vi "Connect PV.vi"(8 "error in (no error)":errorcluster, 10 "PV URL":string, 11 "CS++SVMonitor in":refnum<class "CS++SVMonitor.lvclass">) -> (0 "error out":errorcluster, 3 "CS++SVMonitor out":refnum<class "CS++SVMonitor.lvclass">)   [LabVIEW 2015, in "CS++SVMonitor.lvlib" / "CS++SVMonitor.lvclass"]
doc: "Open connection to process variable."
uses:
  CS++SVMonitor.lvclass
  CS++SVMonitor.lvclass/CS++SVMonitor.ctl
  Libraries/Utilities/CS++Utilities.lvlib
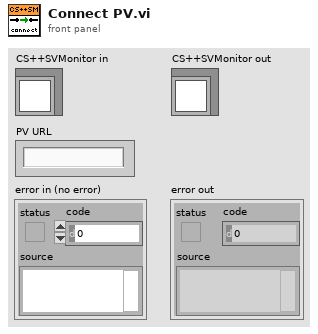
[diagram p1: front panel]
types:
  T1 = cluster{"Read Access":enum8{"Allowed", "Required", "None"}, "Write Access":enum8{"Allowed", "Required", "None"}}
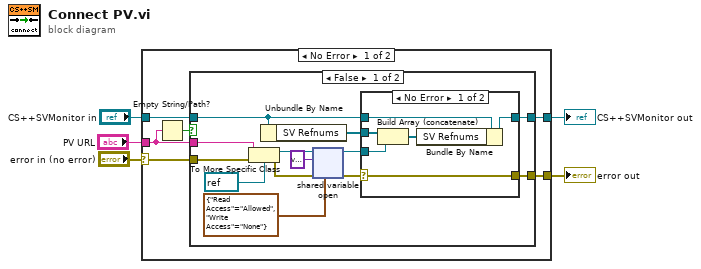
[diagram p0: block diagram]
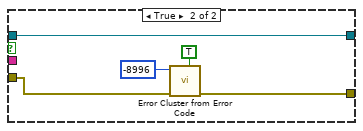
[diagram p3: hidden frame]
diagram:
  n1 = case shown="No Error" "error in (no error)" {
    selector: "error in (no error)" -> [w11 w39]
    tunnel: [w8 w39] -> w2
    tunnel: [w9 w38] -> w3
    tunnel: "CS++SVMonitor in" -> [w10 w38]
    tunnel: "PV URL" -> [w7 _]
    frame No Error {
      n2 = Empty String/Path?(string/path=w7) -> (empty?=w6:bool)
      n3 = case shown="False" w6 {
        tunnel: w11 -> [w19 w35]
        tunnel: w7 -> [w18 _]
        tunnel: w10 -> [w17 w37]
        tunnel: [w16 w37] -> w9
        tunnel: [w13 w34] -> w8
        frame False {
          n4 = To More Specific Class(target class=refnum<k21> refnum ("shared variable refnum in"), reference=w18, error in=w19) -> (specific class reference=w23:refnum<k21>, error out=w22:errorcluster)
          n5 = Unbundle By Name(w17) -> ("SV Refnums"=w15:refnum<k21>[])
          n6 = shared-variable-open(w23, w22, variant ("variant"), T1 {"Read Access"=enum."Allowed", "Write Access"=enum."None"} ("Access (R/W allowed)")) -> (w20:refnum<k21>, w14:errorcluster)
          n7 = case shown="No Error" w14 {
            selector: w14 -> [w25 w31]
            tunnel: w20 -> [w30 _]
            tunnel: w17 -> [w29 w32]
            tunnel: [w28 w32] -> w16
            tunnel: w15 -> [w26 _]
            tunnel: [w25 w31] -> w13
            frame No Error {
              n8 = Build Array (concatenate)(w26, w30) -> (w27:refnum<k21>[])
              n9 = Bundle By Name(cluster=w29, "SV Refnums"=w27) -> (w28:refnum<class "CS++SVMonitor.lvclass">)
            }
            frame Error {
            }
          }
        }
        frame True {
          n10 = call "Error Cluster from Error Code.vi"("is warning? (False)"=TRUE, "Error In"=w35, "Error Code (0)"=-8996 ("error code (no error:0)")) -> ("Error Out"=w34:errorcluster)  [unwired: 8 in]
        }
      }
    }
    frame Error {
    }
  }
  "error out" <- w2
  "CS++SVMonitor out" <- w3
